vi "查询产品ID.vi"(8 "error in (no error)":errorcluster, 11 "芯片编码":string="A001") -> (0 "error out":errorcluster, 2 "产品ID":string, 3 "索引结果":bool)   [LabVIEW 2013]
uses:
  <vilib>/Utility/error.llb/whitespace.ctl
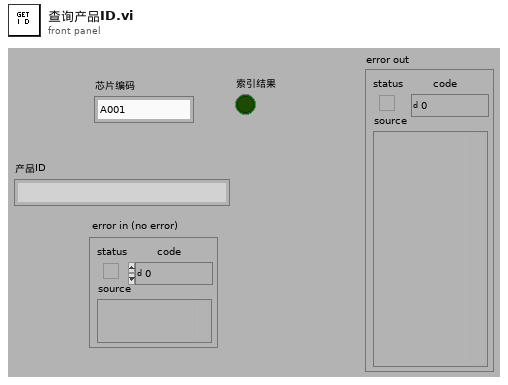
[diagram p1: front panel]
types:
  T1 = typedef "whitespace.ctl" = u16
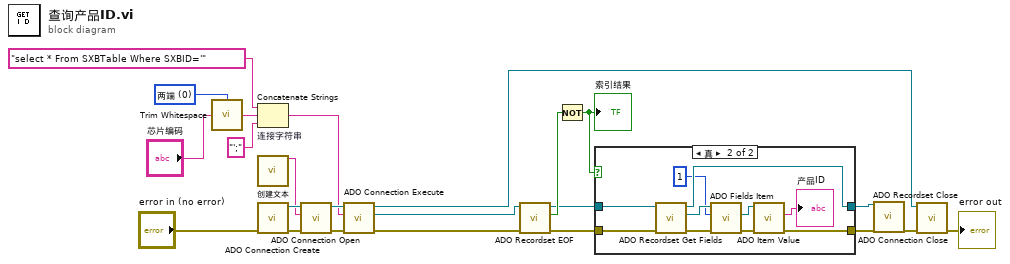
[diagram p0: block diagram]
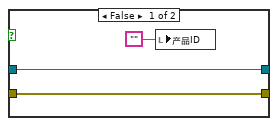
[diagram p2: hidden frame]
diagram:
  w11 = T1 0 items=["两端", "字符串首端", "字符串末端"] ("location (both)")
  n1 = call <vilib>:"Trim Whitespace.vi"("string"="芯片编码", "location (both)"=w11) -> ("trimmed string"=w12:string)
  n2 = Concatenate Strings "连接字符串"("select * From SXBTable Where SXBID='" ("字符串 2"), w12, "';" ("字符串 2")) -> (w10:string)
  n3 = call "创建文本"() -> ("Result"=w1:string)  [unwired: 14 in, 1 out]
  n4 = call "ADO Connection Create.vi"("error in (no error)"="error in (no error)") -> ("error out"=w22:errorcluster, "ADODB._Connection Out"=w23:refnum<k7>)  [unwired: 9 out]
  n5 = call "ADO Connection Open.vi"("error in (no error)"=w22, "ConnectionString"=w1, "ADODB._Connection In"=w23) -> ("error out"=w21:errorcluster, "ADODB._Connection Out"=w20:refnum<k7>)  [unwired: 7 out]
  n6 = call "ADO Connection Execute.vi"("error in (no error)"=w21, "CommandText"=w10, "ADODB._Connection In"=w20) -> ("error out"=w18:errorcluster, "RecordSet"=w19:refnum<k7>, "ADODB._Connection Out"=w15:refnum<k7>)  [unwired: 6 out]
  n7 = call "ADO Recordset EOF.vi"("error in (no error)"=w18, "ADODB._Recordset In"=w19) -> ("error out"=w5:errorcluster, "EOF"=w17:bool, "ADODB._Recordset Out"=w6:refnum<k7>)  [unwired: 7 out]
  n8 = Not(x=w17) -> (.not. x?=w7:bool)
  "索引结果" <- w7
  n9 = case shown="真" w7 {
    tunnel: w6 -> [w25 w36]
    tunnel: w5 -> [w26 w35]
    tunnel: [w25 w34] -> w4
    tunnel: [w26 w28] -> w3
    frame False {
      n10 = local write "产品ID"("") -> ()
    }
    frame True {
      n11 = call "ADO Recordset Get Fields.vi"("error in (no error)"=w35, "ADODB._Recordset In"=w36) -> ("error out"=w27:errorcluster, "Fields Out"=w33:refnum<k7>, "ADODB._Recordset Out"=w34:refnum<k7>)  [unwired: 7 out]
      n12 = call "ADO Fields Item.vi"("error in (no error)"=w27, "Index"=1, "Fields In"=w33) -> ("error out"=w31:errorcluster, "Item Out"=w30:refnum<k7>)  [unwired: 7 out]
      n13 = call "ADO Item Value.vi"("error in (no error)"=w31, "Item In"=w30) -> ("error out"=w28:errorcluster, "Value"=→"产品ID":string)  [unwired: 8 out]
    }
  }
  n14 = call "ADO Recordset Close.vi"("ADODB._Recordset In"=w4, "error in (no error)"=w3) -> ("error out"=w16:errorcluster)  [unwired: 17 out]
  n15 = call "ADO Connection Close.vi"("error in (no error)"=w16, "ADODB._Connection In"=w15) -> ("error out"=→"error out":errorcluster)  [unwired: 9 out]
